vi "changeIntegrationTime.vi"(8 "error in (no error)":errorcluster, 9 "IntegrationTime":dbl=0.002, 10 "ElectrometerController in":refnum<class "ElectrometerController.lvclass">, 11 "ReadyState in":refnum<class "ReadyState.lvclass">) -> (0 "error out":errorcluster, 2 "ElectrometerController out":refnum<class "ElectrometerController.lvclass">, 3 "ReadyState out":refnum<class "ReadyState.lvclass">)   [LabVIEW 2016, in "ReadyState.lvclass"]
uses:
  ReadyState.lvclass
  ElectrometerController/ElectrometerController.lvclass
  ts_electrometeruserevents/Typedefs/StateValue.ctl
  ts_electrometeruserevents/Typedefs/CommandValue.ctl
  ts_electrometeruserevents/Typedefs/PubDataSV.ctl
  ts_sallv_calibrationelectrometer/DataTypes/logevent_IntegrationTime.ctl
  ElectrometerController/ElectrometerController.lvclass/ElectrometerController.ctl
  ts_electrometeruserevents/PubSubDataEvent/PubSubDataEvent.lvclass
  Electrometer.lvclass
  ElectrometerConfiguration/ElectrometerInternalConfiguration.lvclass
  ts_electrometeruserevents/Typedefs/ElectrometerTypedefs.lvlib
  ts_sallv_calibrationelectrometer/SALLV_calibrationElectrometer.lvlib
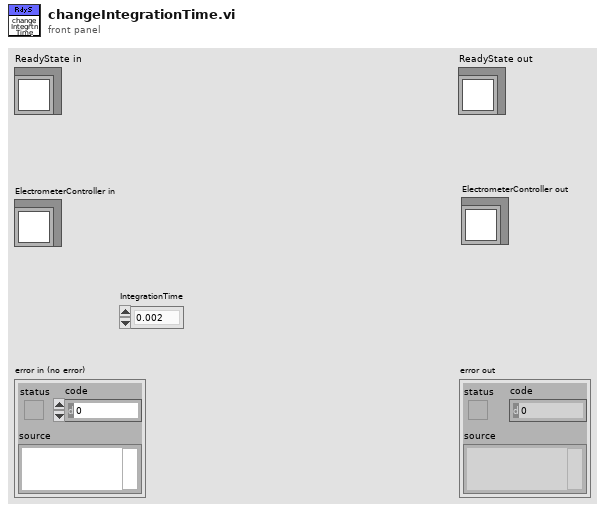
[diagram p1: front panel]
types:
  T1 = cluster{"appliedSettingsMatchStart":bool, "Timestamp":dbl}
  T2 = typedef "ElectrometerTypedefs.lvlib/PubDataSV.ctl" = enum16{"DetailedState", "ErrorCode", "Heartbeat", "LoopTime_ms", "LoopTimeOutOfRange", "RejectedCommand", "SummaryState", "Timestamp", "SettingVersions", "SettingsAppliedSerialConfiguration", "AppliedSettingsMatchStart", "InternalState", "Intensity", "MeasureType", "MeasureRange", "DigitalFilterChange", "IntensityReq", "IntegrationTime", "SettingsAppliedReadingSettings"}
  T3 = typedef "SALLV_calibrationElectrometer.lvlib/logevent_IntegrationTime.ctl" = cluster{"electtId":i16, "intTime":sgl, "priority":i32}
  T4 = typedef "ElectrometerTypedefs.lvlib/CommandValue.ctl" = enum16{"ClearError", "Disable", "Enable", "Exit", "GoToStandby", "OnHeartbeat", "OnIncomingMessagingError", "OnInterrupt", "Start", "SetDigitalFilter", "StartScan", "StartScanDt", "StartScanReachIntensity", "StopScan", "SetIntegrationTime", "PerformZeroCalib", "SetRange", "SetMode", "Power"}
  T5 = typedef "ElectrometerTypedefs.lvlib/StateValue.ctl" = enum16{"", "DisabledState", "EnabledState", "FaultState", "OffState", "StandbyState", "ReadyState", "ConfiguringState", "ManualReadingState", "UntilIntensityReadingState", "SetDurationReadingState", "BufferReadingState"}
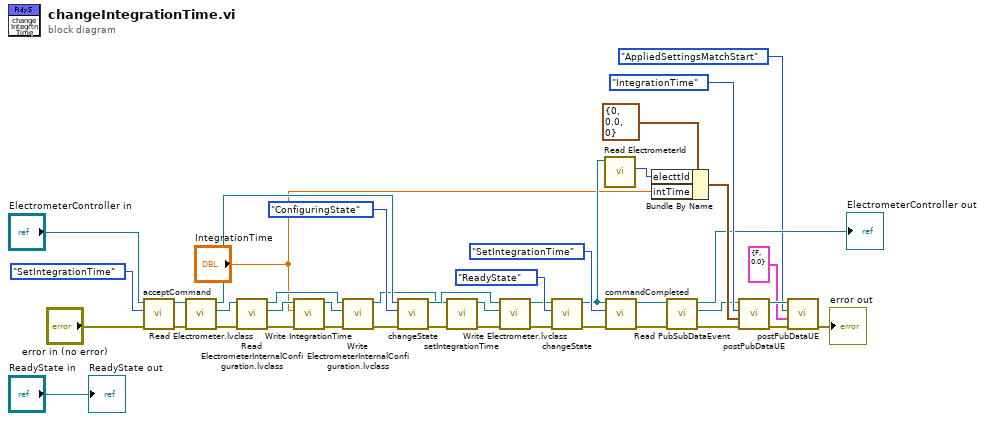
[diagram p0: block diagram]
diagram:
  n1 = call "acceptCommand.vi"("error in (no error)"="error in (no error)", "CommandValue"=CommandValue."SetIntegrationTime", "ElectrometerController in"="ElectrometerController in") -> ("error out"=w25:errorcluster, "ElectrometerController out"=w26:refnum<class "ElectrometerController.lvclass">)  [unwired: 7 in]
  n2 = call-dynamic "Read Electrometer.lvclass.vi"("error in (no error)"=w25, "ElectrometerController in"=w26) -> ("error out"=w31:errorcluster, "Electrometer.lvclass"=w32:refnum<class "Electrometer.lvclass">, "ElectrometerController out"=w19:refnum<class "ElectrometerController.lvclass">)  [unwired: 7 in]
  n3 = call-dynamic "Read ElectrometerInternalConfiguration.lvclass.vi"("error in (no error)"=w31, "Electrometer in"=w32) -> ("error out"=w30:errorcluster, "ElectrometerInternalConfiguration.lvclass"=w29:refnum<class "ElectrometerInternalConfiguration.lvclass">, "Electrometer out"=w33:refnum<class "Electrometer.lvclass">)  [unwired: 7 in]
  n4 = call-dynamic "Write IntegrationTime.vi"("error in (no error)"=w30, "IntegrationTime"="IntegrationTime", "ElectrometerInternalConfiguration in"=w29) -> ("error out"=w27:errorcluster, "ElectrometerInternalConfiguration out"=w28:refnum<class "ElectrometerInternalConfiguration.lvclass">)  [unwired: 7 in]
  n5 = call-dynamic "Write ElectrometerInternalConfiguration.lvclass.vi"("error in (no error)"=w27, "ElectrometerInternalConfiguration.lvclass"=w28, "Electrometer in"=w33) -> ("error out"=w18:errorcluster, "Electrometer out"=w17:refnum<class "Electrometer.lvclass">)  [unwired: 7 in]
  n6 = call "changeState.vi"("error in (no error)"=w18, "StateValue"=StateValue."ConfiguringState", "ElectrometerController in"=w19) -> ("error out"=w41:errorcluster, "ElectrometerController out"=w22:refnum<class "ElectrometerController.lvclass">)  [unwired: 7 in]
  n7 = call "setIntegrationTime.vi"("error in (no error)"=w41, "Electrometer in"=w17) -> ("error out"=w24:errorcluster, "Electrometer out"=w23:refnum<class "Electrometer.lvclass">)  [unwired: 8 in]
  n8 = call-dynamic "Write Electrometer.lvclass.vi"("error in (no error)"=w24, "Electrometer.lvclass"=w23, "ElectrometerController in"=w22) -> ("error out"=w20:errorcluster, "ElectrometerController out"=w21:refnum<class "ElectrometerController.lvclass">)  [unwired: 7 in]
  n9 = call "changeState.vi"("error in (no error)"=w20, "StateValue"=StateValue."ReadyState", "ElectrometerController in"=w21) -> ("error out"=w35:errorcluster, "ElectrometerController out"=w3:refnum<class "ElectrometerController.lvclass">)  [unwired: 7 in]
  n10 = call-dynamic "Read ElectrometerId.vi"("ElectrometerController in"=w3) -> ("ElectrometerId"=w2:enum16{"", "ID1", "ID2"})  [unwired: 8 in, 2 out]
  n11 = call "commandCompleted.vi"("error in (no error)"=w35, "CommandValue"=CommandValue."SetIntegrationTime", "ElectrometerController in"=w3) -> ("error out"=w14:errorcluster, "ElectrometerController out"=w15:refnum<class "ElectrometerController.lvclass">)  [unwired: 7 in]
  n12 = Bundle By Name(cluster=T3 {"electtId"=0, "intTime"=0.0, "priority"=0} ("logevent_IntegrationTime"), "electtId"=w2, "intTime"="IntegrationTime") -> (w12:T3)
  n13 = call "Read PubSubDataEvent.vi"("error in (no error)"=w14, "ElectrometerController in"=w15) -> ("error out"=w11:errorcluster, "PubSubDataEvent.lvclass"=w10:refnum<class "PubSubDataEvent.lvclass">, "ElectrometerController out"=→"ElectrometerController out":refnum<class "ElectrometerController.lvclass">)  [unwired: 7 in]
  n14 = call "postPubDataUE.vi"("error in (no error)"=w11, "value"=w12, "pubDataSV"=PubDataSV."IntegrationTime", "PubSubDataEvent in"=w10) -> ("error out"=w5:errorcluster, "PubSubDataEvent out"=w8:refnum<class "PubSubDataEvent.lvclass">)  [unwired: 6 in]
  n15 = call "postPubDataUE.vi"("error in (no error)"=w5, "value"=T1 {"appliedSettingsMatchStart"=FALSE, "Timestamp"=0.0} ("event data"), "pubDataSV"=PubDataSV."AppliedSettingsMatchStart", "PubSubDataEvent in"=w8) -> ("error out"=→"error out":errorcluster)  [unwired: 6 in, 1 out]
  "ReadyState out" <- "ReadyState in"
